vi "零件加工（简单工厂）.vi"() -> ()   [LabVIEW 2011]
panel:
  out "Output":string
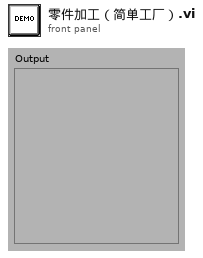
[diagram p1: front panel]
types:
  T1 = typedef "简单加工类工厂.lvclass/加工方法.ctl" = enum16{"车削", "铣削", "钻削"}
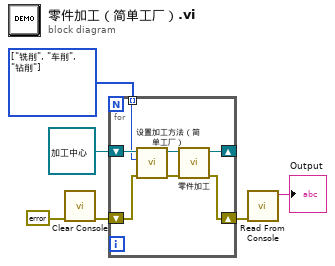
[diagram p0: block diagram]
diagram:
  w3 = T1[] [enum."铣削", enum."车削", enum."钻削"] items=["车削", "铣削", "钻削"]
  n1 = call "Clear Console.vi"("error in (no error)"=errorcluster {"status"=FALSE, "code"=0, "source"=""} ("error out")) -> ("error out"=w1:errorcluster)  [unwired: 10 in]
  n2 = for {
    shift-right: [w13] -> _
    shift-left: refnum<class "加工中心.lvclass"> refnum ("加工中心.lvclass") -> [w11]
    shift-right: [w12] -> w5
    shift-left: w1 -> [w9]
    tunnel: w3 -> [w7] mode=indexing
    n3 = call "设置加工方法（简单工厂）.vi"("error in (no error)"=w9, "加工方法"=w7, "加工中心 输入"=w11) -> ("error out"=w8:errorcluster, "加工中心 输出"=w10:refnum<class "加工中心.lvclass">)  [unwired: 7 in]
    n4 = call "零件加工.vi"("error in (no error)"=w8, "加工中心 输入"=w10) -> ("error out"=w12:errorcluster, "加工中心 输出"=w13:refnum<class "加工中心.lvclass">)  [unwired: 8 in]
  }
  n5 = call "Read From Console.vi"("error in (no error)"=w5) -> ("Output"=→"Output":string)  [unwired: 9 in, 1 out]
